vi "Set Card Read.vi"(8 "error in (no error)":errorcluster, 10 "Card read":bool, 11 "ATM Controller in":refnum<class "ATM Controller.lvclass">) -> (0 "error out":errorcluster, 3 "ATM Controller out":refnum<class "ATM Controller.lvclass">)   [LabVIEW 2019, in "ATM Controller.lvlib" / "ATM Controller.lvclass"]
uses:
  ATM Controller.lvclass
  ATM Controller.lvclass/ATM Controller.ctl
  Sim Display Console Actor/Sim Display Console Actor Messages/Write Card Read Msg/Write Card Read Msg.lvclass/Write Card Read Msg.ctl
  <vilib>/ActorFramework/Message Enqueuer/Message Enqueuer.lvclass/Message Enqueuer.ctl
  <vilib>/ActorFramework/Message Enqueuer/Enqueue.vi
  Sim Display Console Actor/Sim Display Console Actor Messages/Write Card Read Msg/Write Card Read Msg.lvclass
  C:/Program Files (x86)/National Instruments/LabVIEW 2019/vi.lib/ActorFramework/Message/Message.lvclass
  <vilib>/ActorFramework/Message Priority Queue/Priority Enqueue.vi
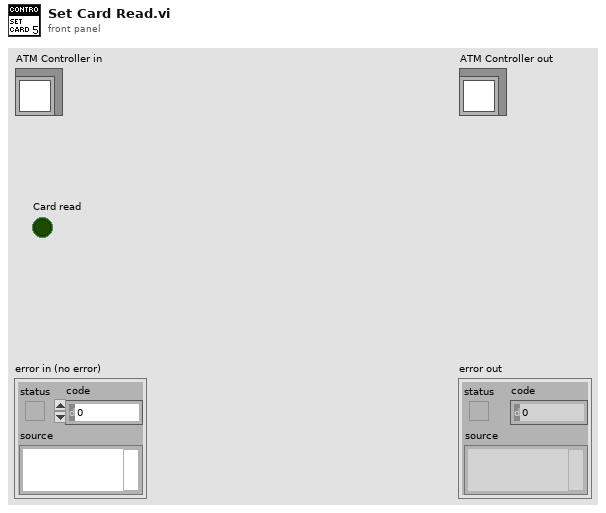
[diagram p1: front panel]
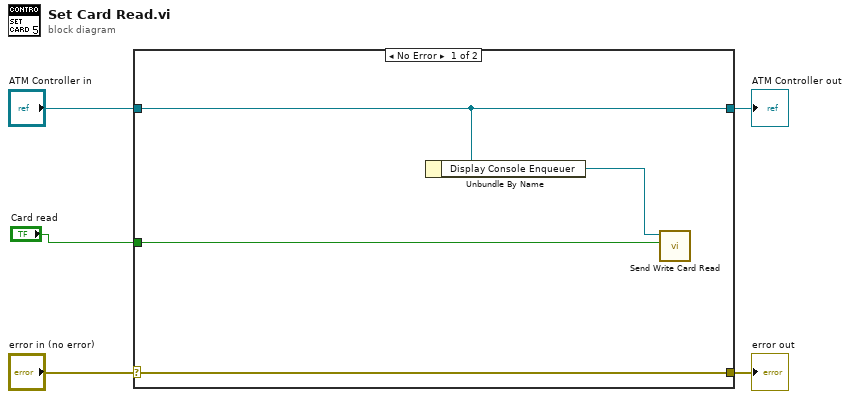
[diagram p0: block diagram]
diagram:
  n1 = case shown="No Error" "error in (no error)" {
    selector: "error in (no error)" -> [w9 w11]
    tunnel: [w9 w11] -> w4
    tunnel: [w8 w10] -> w2
    tunnel: "ATM Controller in" -> [w8 w10]
    tunnel: "Card read" -> [w6 _]
    frame No Error {
      n2 = Unbundle By Name(w8) -> ("Display Console Enqueuer"=w7:refnum<class "Message Enqueuer.lvclass">)
      n3 = call "Send Write Card Read.vi"("Card read"=w6, "Message Enqueuer"=w7) -> ()  [unwired: 8 in, 2 out]
    }
    frame Error {
    }
  }
  "error out" <- w4
  "ATM Controller out" <- w2
